vi "Find Repository Root.vi"(8 "error in":errorcluster, 11 "Package Source Folder":path) -> (0 "error out":errorcluster, 3 "repository path":path)   [LabVIEW 2019]
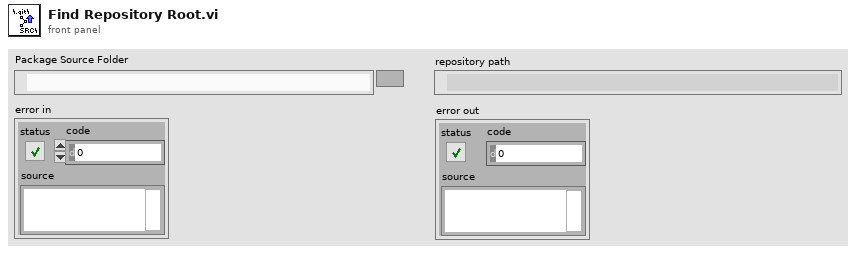
[diagram p1: front panel]
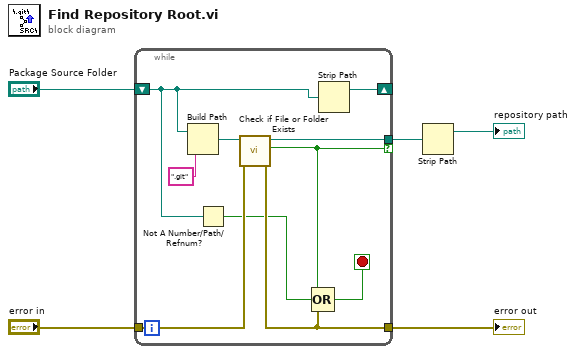
[diagram p0: block diagram]
diagram:
  n1 = while {
    tunnel: [w13] -> w1
    tunnel: "error in" -> [w12]
    shift-right: [w15] -> _
    shift-left: "Package Source Folder" -> [w8]
    tunnel: [w9] -> w3 if=w6
    stop <- w14 stop-if-true
    n2 = Build Path(base path=w8, name or relative path=".git" ("pattern")) -> (appended path=w10:path)
    n3 = Not A Number/Path/Refnum?(number/path/refnum=w8) -> (NaN/Path/Refnum?=w7:bool)
    n4 = call <vilib>:"Check if File or Folder Exists.vi"("error in (no error)"=w12, "path"=w10) -> ("error out"=w13:errorcluster, "file or folder exists?"=w6:bool, "dup path"=w9:path)  [unwired: 7 in]
    n5 = Compound Arithmetic op=OR(w6, w7, w13) -> (w14:bool)
    n6 = Strip Path(path=w8) -> (stripped path=w15:path)  [unwired: 1 out]
  }
  "error out" <- w1
  n7 = Strip Path(path=w3) -> (stripped path=→"repository path":path)  [unwired: 1 out]
